vi "CreateServer.vi"() -> (3 "gRPCid":T1)   [LabVIEW 2019, in "gprc-support.lvlib"]
uses:
  gprc-support.lvlib
  grpcId.ctl
  home/lvuser/liblabview_grpc_server.so
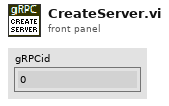
[diagram p1: front panel]
types:
  T1 = typedef "gprc-support.lvlib/grpcId.ctl" = u64
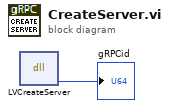
[diagram p0: block diagram]
diagram:
  n1 = dll-call lib="home/lvuser/liblabview_grpc_server.so" fn="LVCreateServer"() -> ("gRPCid"=→"gRPCid":T1)  [unwired: 5 in, 2 out]
